vi "get SA province data.vi"() -> (1 "populations":i32[](array[numeric]), 2 "SA province names":string[](array[string]), 3 "SA data":T1)   [LabVIEW 2019]
uses:
  Globals.vi
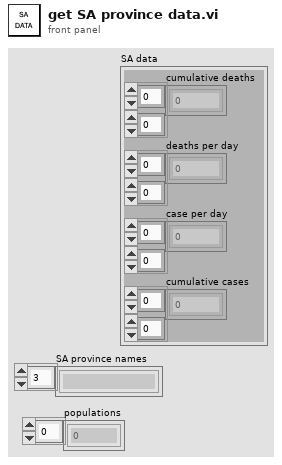
[diagram p1: front panel]
types:
  T1 = cluster{"cumulative deaths":i32[][], "deaths per day":i32[][], "case per day":i32[][], "cumulative cases":i32[][]}
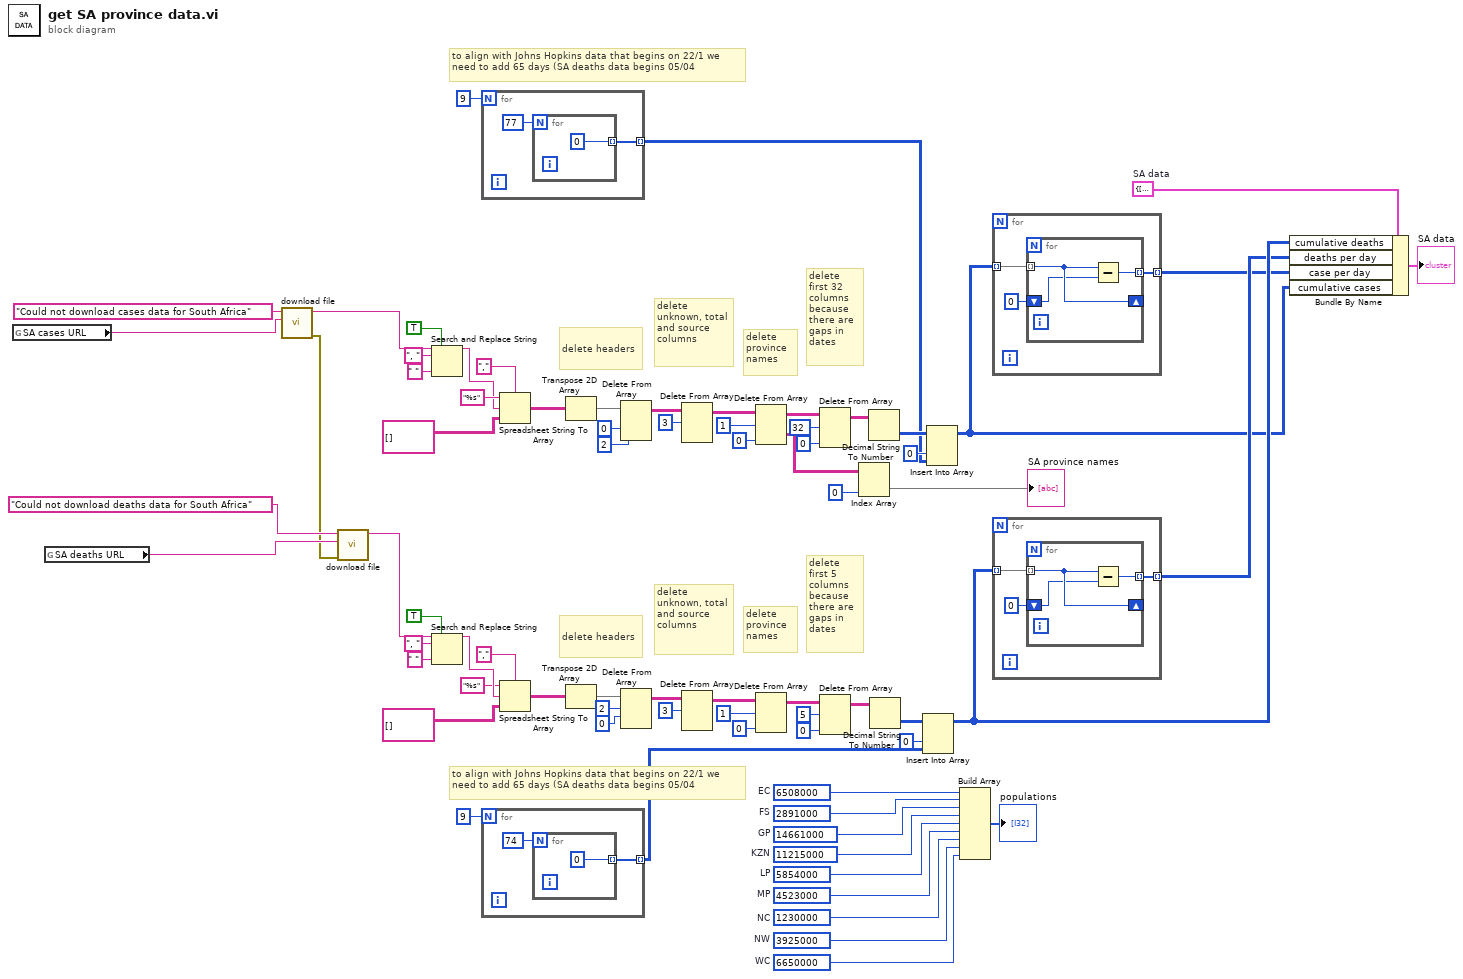
[diagram p0: block diagram]
diagram:
  w13 = T1 {"cumulative deaths"=[], "deaths per day"=[], "case per day"=[], "cumulative cases"=[]}  # SA data
  w30 = 6650000  # WC
  w31 = 3925000  # NW
  w32 = 1230000  # NC
  w33 = 4523000  # MP
  w34 = 5854000  # LP
  w35 = 11215000  # KZN
  w36 = 14661000  # GP
  w37 = 2891000  # FS
  w38 = 6508000  # EC
  # "to align with Johns Hopkins data that begins on 22/1 we need to add 65 days (SA deaths data begins 05/04"
  # "delete first 32 columns because there are gaps in dates"
  # "delete first 5 columns because there are gaps in dates"
  # "delete province names"
  # "delete province names"
  # "to align with Johns Hopkins data that begins on 22/1 we need to add 65 days (SA deaths data begins 05/04"
  # "delete unknown, total and source columns"
  # "delete headers"
  # "delete unknown, total and source columns"
  # "delete headers"
  n1 = global read "Globals.vi" "SA cases URL"() -> (w6:string)
  n2 = global read "Globals.vi" "SA deaths URL"() -> (w4:string)
  n3 = call "download file.vi"("URL"=w6, "Error message"="Could not download cases data for South Africa") -> ("error out"=w1:errorcluster, "downloaded file"=w7:string)  [unwired: 8 in]
  n4 = call "download file.vi"("error in (no error)"=w1, "URL"=w4, "Error message"="Could not download deaths data for South Africa") -> ("downloaded file"=w2:string)  [unwired: 7 in, 1 out]
  n5 = Search and Replace String(replace all?=TRUE ("replace all? (F)"), input string=w7, search string=", ", replace string=" " ("replace string (\"\")")) -> (result string=w68:string)  [unwired: 4 in, 3 out]
  n6 = Search and Replace String(replace all?=TRUE ("replace all? (F)"), input string=w2, search string=", ", replace string=" " ("replace string (\"\")")) -> (result string=w46:string)  [unwired: 4 in, 3 out]
  n7 = for {
    N: 9 -> [_]
    tunnel: [w75] -> w14 mode=indexing
    n8 = for {
      N: 77 -> [_]
      tunnel: [0] -> w75 mode=indexing
    }
  }
  n9 = for {
    N: 9 -> [_]
    tunnel: [w78] -> w25 mode=indexing
    n10 = for {
      N: 74 -> [_]
      tunnel: [0] -> w78 mode=indexing
    }
  }
  n11 = Spreadsheet String To Array(delimiter (Tab)=",", format string="%s", spreadsheet string=w68, array type (2D Dbl)=string[][] []) -> (array=w67:string[][])
  n12 = Spreadsheet String To Array(delimiter (Tab)=",", format string="%s", spreadsheet string=w46, array type (2D Dbl)=string[][] []) -> (array=w47:string[][])
  n13 = Transpose 2D Array(2D array=w67) -> (transposed array=w66:string[][])
  n14 = Transpose 2D Array(2D array=w47) -> (transposed array=w48:string[][])
  n15 = Delete From Array(array=w66, length=2, index (row)=0) -> (array with subset deleted=w63:string[][])  [unwired: 1 in, 1 out]
  n16 = Delete From Array(array=w48, length=2, index (row)=0) -> (array with subset deleted=w51:string[][])  [unwired: 1 in, 1 out]
  n17 = Delete From Array(array=w63, length=3) -> (array with subset deleted=w61:string[][])  [unwired: 2 in, 1 out]
  n18 = Delete From Array(array=w51, length=3) -> (array with subset deleted=w53:string[][])  [unwired: 2 in, 1 out]
  n19 = Delete From Array(array=w61, length=1, index (col)=0 ("disabled index (col)")) -> (deleted portion=w58:string[][], array with subset deleted=w17:string[][])  [unwired: 1 in]
  n20 = Delete From Array(array=w53, length=1, index (col)=0 ("disabled index (col)")) -> (array with subset deleted=w23:string[][])  [unwired: 1 in, 1 out]
  n21 = Delete From Array(array=w17, length=32, index (col)=0 ("disabled index (col)")) -> (array with subset deleted=w16:string[][])  [unwired: 1 in, 1 out]
  n22 = Delete From Array(array=w23, length=5, index (col)=0 ("disabled index (col)")) -> (array with subset deleted=w22:string[][])  [unwired: 1 in, 1 out]
  n23 = Index Array(array=w58, index (col)=0 ("disabled index (col)")) -> (element=→"SA province names":string[])  [unwired: 1 in]
  n24 = Decimal String To Number(string=w16) -> (number=w27:i32[][])  [unwired: 2 in, 1 out]
  n25 = Decimal String To Number(string=w22) -> (number=w39:i32[][])  [unwired: 2 in, 1 out]
  n26 = Insert Into Array(array=w39, index (col)=0 ("disabled index (col)"), new element=w25) -> (w12:i32[][])  [unwired: 1 in]
  n27 = Insert Into Array(array=w27, index (col)=0 ("disabled index (col)"), new element=w14) -> (w9:i32[][])  [unwired: 1 in]
  n28 = Build Array(w38, w37, w36, w35, w34, w33, w32, w31, w30) -> (→"populations":i32[])
  n29 = for {
    tunnel: [w82] -> w10 mode=indexing
    tunnel: w9 -> [w81] mode=indexing
    n30 = for {
      tunnel: w81 -> [w86] mode=indexing
      shift-right: [w86] -> _
      shift-left: 0 -> [w85]
      tunnel: [w84] -> w82 mode=indexing
      n31 = Subtract(x=w86, y=w85) -> (x-y=w84:i32)
    }
  }
  n32 = for {
    tunnel: [w88] -> w11 mode=indexing
    tunnel: w12 -> [w87] mode=indexing
    n33 = for {
      tunnel: w87 -> [w92] mode=indexing
      shift-right: [w92] -> _
      shift-left: 0 -> [w91]
      tunnel: [w90] -> w88 mode=indexing
      n34 = Subtract(x=w92, y=w91) -> (x-y=w90:i32)
    }
  }
  n35 = Bundle By Name(cluster=w13, "cumulative deaths"=w12, "deaths per day"=w11, "case per day"=w10, "cumulative cases"=w9) -> (→"SA data":T1)
